vi "chooseOffensivePlay.vi"(8 "error in (no error)":errorcluster, 11 "Game in":refnum<class "Game.lvclass">) -> (0 "error out":errorcluster, 3 "Game out":refnum<class "Game.lvclass">)   [LabVIEW 2023, in "Game.lvclass"]
uses:
  Game.lvclass
  Referee_class/command_interpreted.ctl
  Game.lvclass/Game.ctl
  Team_class/Team.lvclass/Team.ctl
  Referee_class/Referee.lvclass/Referee.ctl
  StopOffensivePlay_class/StopOffensivePlay.lvclass
  PreparePenaltyEnemyPlay_class/PreparePenaltyEnemyPlay.lvclass
  EnemyPossessionAtEnemyFieldPlay_class/EnemyPossessionAtEnemyFieldPlay.lvclass
  EnemyPossessionAtOurFieldPlay_class/EnemyPossessionAtOurFieldPlay.lvclass
  PreparePenaltyAllyPlay_class/PreparePenaltyAllyPlay.lvclass
  KickPenaltyAllyPlay_class/KickPenaltyAllyPlay.lvclass
  PrepareKickoffAllyPlay_class/PrepareKickoffAllyPlay.lvclass
  PrepareKickoffEnemyPlay_class/PrepareKickoffEnemyPlay.lvclass
  SimplePass_class/SimplePass.lvclass
  PreparePassPlay_class/PreparePassPlay.lvclass
  PrepareRollToPassPlay_class/PrepareRollToPassPlay.lvclass
  PrepareDoublePassPlay_class/PrepareDoublePassPlay.lvclass
  PassToStriker_class/PassToStriker.lvclass
  C:/Users/roboi/Downloads/VSS_AI-Larc2023/Play_class/Play.lvclass
  PassTo2ndStriker_class/PassTo2ndStriker.lvclass
  TableWithStrikerPlay_class/TableWithStrikerPlay.lvclass
  TableWith2ndStrikerPlay_class/TableWith2ndStrikerPlay.lvclass
  DirectKickPlay_class/DirectKickPlay.lvclass
  DirectEnemyPlay_class/DirectEnemyPlay.lvclass
  NormalGamePlay_class/NormalGamePlay.lvclass
  TestPlay_class/TestPlay.lvclass
  BallOutOfFieldPlay_class/BallOutOfFieldPlay.lvclass
  Team_class/OffensivePlay.ctl
  Utilities_class/Utilities.lvclass
  Read OffensiveTeam.vi
  Read Referee.vi
  Referee_class/Read command_interpreted.vi
  Team_class/Read OffensivePlay.vi
  Team_class/Write OffensivePlay.vi
  Write OffensiveTeam.vi
  Ally_class/Ally.lvclass
  C:/Users/roboi/Downloads/VSS_AI-Larc2023/Team_class/Team.lvclass
  Referee_class/Referee.lvclass
  PassPlay_class/PassPlay.lvclass
  Play_class/Play.lvclass
panel:
  in  "Game in":refnum<class "Game.lvclass">
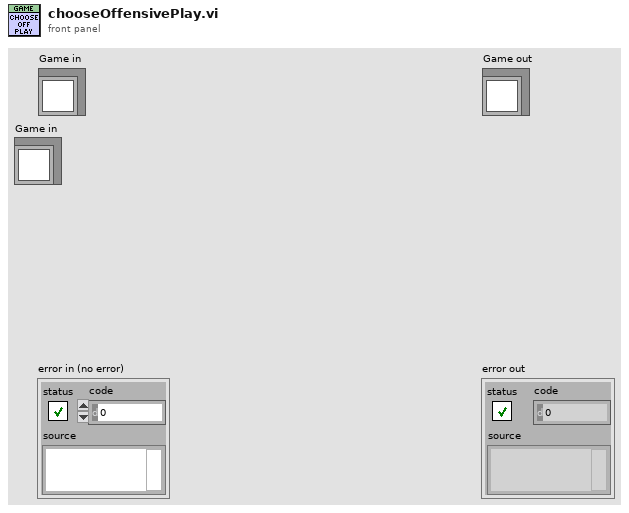
[diagram p1: front panel]
types:
  T1 = typedef "OffensivePlay.ctl" = enum16{"TableWithStriker", "TableWith2ndStrikerPlay", "PrepareDoublePass", "PrepareRollToPass", "SimplePass", "PreparePass", "PassToStriker", "BallOutOfField", "PassTo2ndStriker", "StopOffensive", "Prepare Penalty Enemy", "EnemyPossessionAtEnemyField", "EnemyPossesionAtOurField", "TestPlay", "PreparePenaltyAlly", "KickPenaltyAlly", "PrepareKickoffAlly", "PrepareKickoffEnemy", "IndirectEnemy", "DirectEnemy", "NormalGame", "DirectKick", "Pass", "Halt", "Timeout", "PassPlay", "PenaltyEnemy"}
  T2 = typedef "command_interpreted.ctl" = enum16{"Goal Ally", "Goal Enemy", "Ball Placement Enemy", "Ball Placement Ally", "Normal Half Time", "Extra Time  Break", "Extra Half Time", "None", "Post Game", "PKA Normal Start", "Prepare Kickoff Ally", "PKE Normal Start", "Prepare Kickoff Enemy", "Force Start", "Halt", "Timeout", "Prepare Penalty Ally", "Prepare Penalty Enemy", "PPA NormalStart", "PPE Normal Start", "Indirect Free Ally", "Direct Free Enemy", "Direct Free Ally", "Indirect Free Enemy", "Stop"}
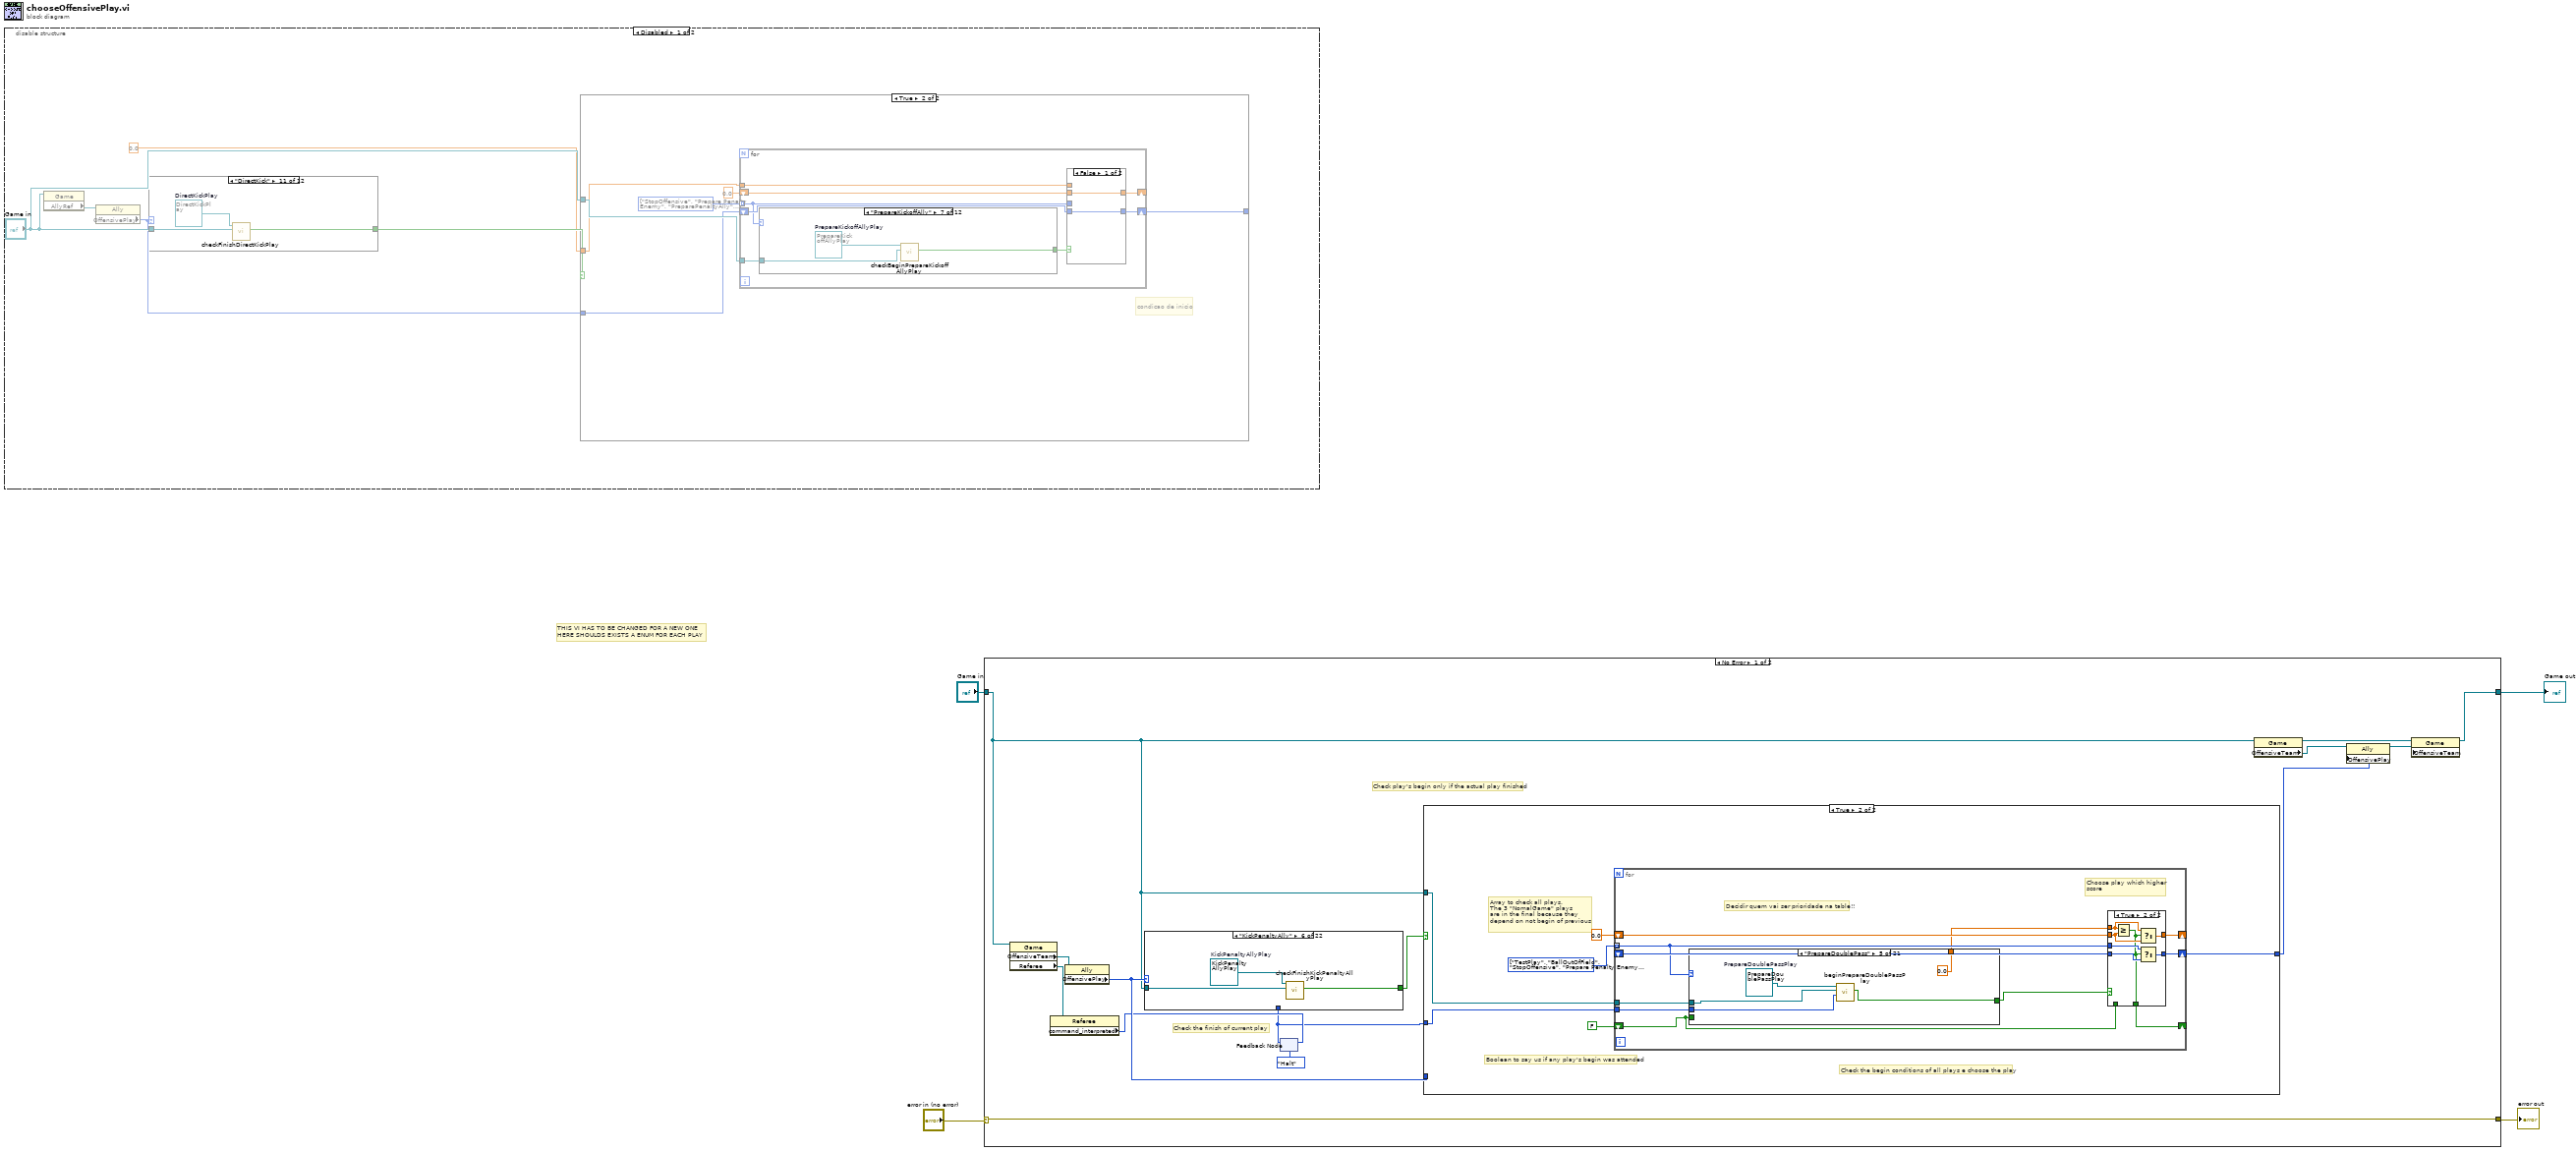
[diagram p0: block diagram]
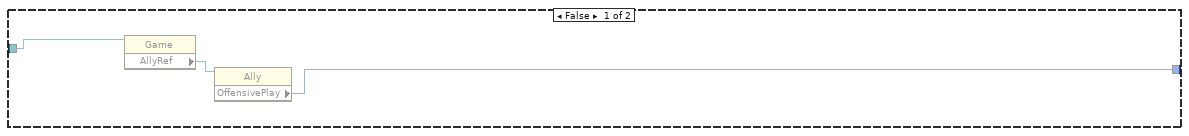
[diagram p2: hidden frame]
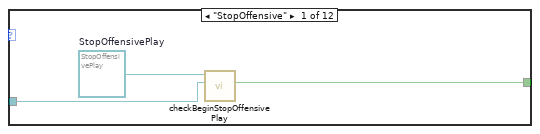
[diagram p3: hidden frame]
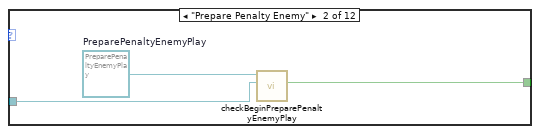
[diagram p4: hidden frame]
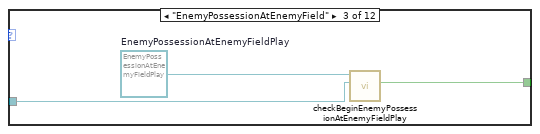
[diagram p5: hidden frame]
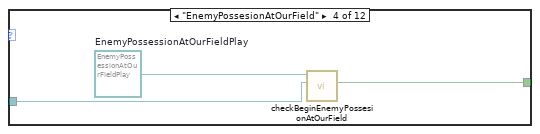
[diagram p6: hidden frame]
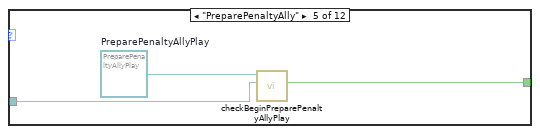
[diagram p7: hidden frame]
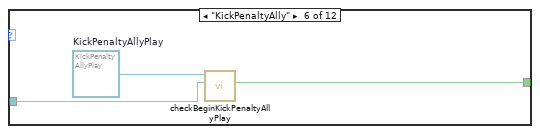
[diagram p8: hidden frame]
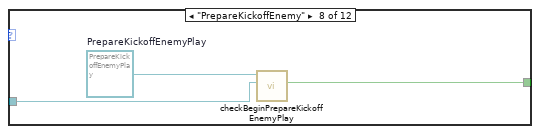
[diagram p9: hidden frame]
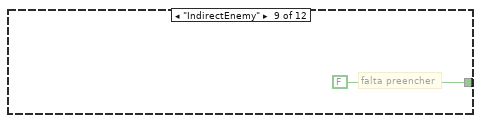
[diagram p10: hidden frame]
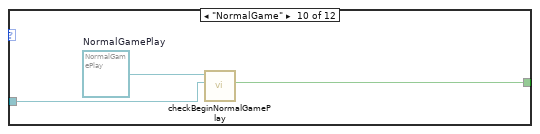
[diagram p11: hidden frame]
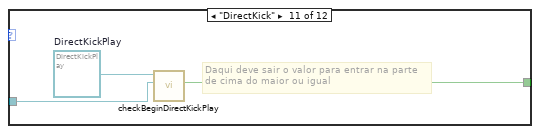
[diagram p12: hidden frame]
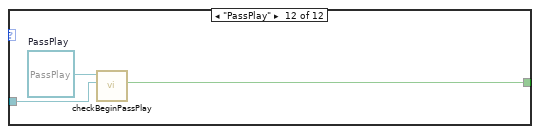
[diagram p13: hidden frame]
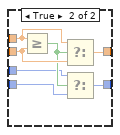
[diagram p14: hidden frame]
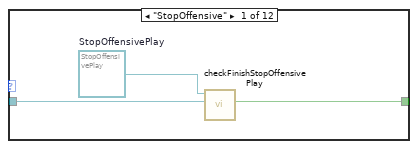
[diagram p15: hidden frame]
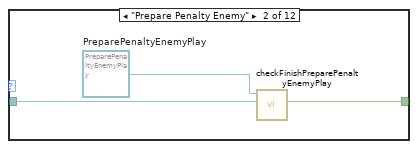
[diagram p16: hidden frame]
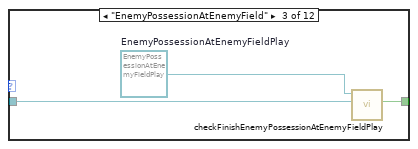
[diagram p17: hidden frame]
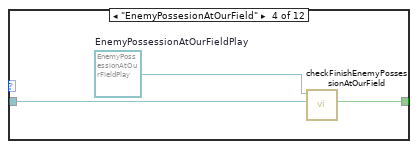
[diagram p18: hidden frame]
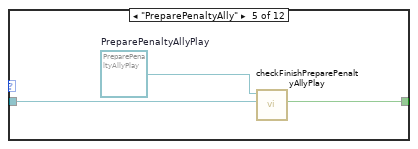
[diagram p19: hidden frame]
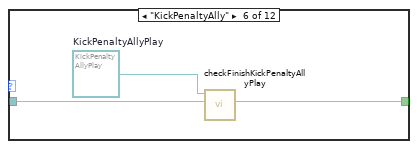
[diagram p20: hidden frame]
diagram:
  # "THIS VI HAS TO BE CHANGED FOR A NEW ONE\nHERE SHOULDS EXISTS A ENUM FOR EACH PLAY"
  n1 = disable-structure shown="Disabled" {
    frame Disabled {
      n2 = property class="Game"(reference="Game in") -> ("AllyRef"=w7:refnum<class "Ally.lvclass">)  [unwired: 1 in, 2 out]
      n3 = property class="Ally"(reference=w7) -> ("OffensivePlay"=w6:T1)  [unwired: 1 in, 2 out]
      n4 = case shown="\"DirectKick\"" w6 {
        tunnel: [w72 w74 w77 w80 w83 w86 w89 w92 FALSE w96 w99 w102] -> w9
        tunnel: "Game in" -> [w70 w75 w78 w81 w84 w87 w90 w93 _ w97 w100 w103]
        frame "StopOffensive" {
          w71 = refnum<class "StopOffensivePlay.lvclass"> refnum  # StopOffensivePlay
          n5 = call "checkFinishStopOffensivePlay.vi"("Game"=w70, "StopOffensivePlay in"=w71) -> ("Boolean"=w72:bool)  [unwired: 7 in, 2 out]
        }
        frame "Prepare Penalty Enemy" {
          w73 = refnum<class "PreparePenaltyEnemyPlay.lvclass"> refnum  # PreparePenaltyEnemyPlay
          n6 = call "checkFinishPreparePenaltyEnemyPlay.vi"("Game"=w75, "PreparePenaltyEnemyPlay in"=w73) -> ("Boolean"=w74:bool)  [unwired: 7 in, 2 out]
        }
        frame "EnemyPossessionAtEnemyField" {
          w76 = refnum<class "EnemyPossessionAtEnemyFieldPlay.lvclass"> refnum  # EnemyPossessionAtEnemyFieldPlay
          n7 = call "checkFinishEnemyPossessionAtEnemyFieldPlay.vi"("Game"=w78, "EnemyPossessionAtEnemyFieldPlay in"=w76) -> ("Boolean"=w77:bool)  [unwired: 7 in, 2 out]
        }
        frame "EnemyPossesionAtOurField" {
          w79 = refnum<class "EnemyPossessionAtOurFieldPlay.lvclass"> refnum  # EnemyPossessionAtOurFieldPlay
          n8 = call "checkFinishEnemyPossessionAtOurField.vi"("Game"=w81, "EnemyPossessionAtOurFieldPlay in"=w79) -> ("Boolean"=w80:bool)  [unwired: 7 in, 2 out]
        }
        frame "PreparePenaltyAlly" {
          w82 = refnum<class "PreparePenaltyAllyPlay.lvclass"> refnum  # PreparePenaltyAllyPlay
          n9 = call "checkFinishPreparePenaltyAllyPlay.vi"("Game"=w84, "PreparePenaltyAllyPlay in"=w82) -> ("Boolean"=w83:bool)  [unwired: 7 in, 2 out]
        }
        frame "KickPenaltyAlly" {
          w85 = refnum<class "KickPenaltyAllyPlay.lvclass"> refnum  # KickPenaltyAllyPlay
          n10 = call "checkFinishKickPenaltyAllyPlay.vi"("Game"=w87, "KickPenaltyAllyPlay in"=w85) -> ("Boolean"=w86:bool)  [unwired: 7 in, 2 out]
        }
        frame "PrepareKickoffAlly" {
          w88 = refnum<class "PrepareKickoffAllyPlay.lvclass"> refnum  # PrepareKickoffAllyPlay
          n11 = call "checkFinishPrepareKickoffAllyPlay.vi"("Game"=w90, "PrepareKickoffAllyPlay in"=w88) -> ("Boolean"=w89:bool)  [unwired: 7 in, 2 out]
        }
        frame "PrepareKickoffEnemy" {
          w91 = refnum<class "PrepareKickoffEnemyPlay.lvclass"> refnum  # PrepareKickoffEnemyPlay
          n12 = call "checkFinishPrepareKickoffEnemyPlay.vi"("Game"=w93, "PrepareKickoffEnemyPlay in"=w91) -> ("Boolean"=w92:bool)  [unwired: 7 in, 2 out]
        }
        frame "IndirectEnemy" {
          # "falta preencher"
        }
        frame "NormalGame" {
          w95 = refnum<class "NormalGamePlay.lvclass"> refnum  # NormalGamePlay
          n13 = call "checkFinishNormalGamePlay.vi"("Game"=w97, "NormalGamePlay in"=w95) -> ("Boolean"=w96:bool)  [unwired: 7 in, 2 out]
        }
        frame "DirectKick" {
          w98 = refnum<class "DirectKickPlay.lvclass"> refnum  # DirectKickPlay
          n14 = call "checkFinishDirectKickPlay.vi"("Game"=w100, "DirectKickPlay in"=w98) -> ("Boolean"=w99:bool)  [unwired: 7 in, 2 out]
        }
        frame "PassPlay" {
          w101 = refnum<class "PassPlay.lvclass"> refnum  # PassPlay
          n15 = call "checkFinishPassPlay.vi"("Game"=w103, "PassPlay in"=w101) -> ("Boolean"=w102:bool)  [unwired: 7 in, 2 out]
        }
      }
      n16 = case shown="True" w9 {
        tunnel: "Game in" -> [w12 w17]
        tunnel: w6 -> [_ w16]
        tunnel: 0.0 -> [_ w14]
        tunnel: [w10 w13] -> _
        frame False {
          n17 = property class="Game"(reference=w12) -> ("AllyRef"=w11:refnum<class "Ally.lvclass">)  [unwired: 1 in, 2 out]
          n18 = property class="Ally"(reference=w11) -> ("OffensivePlay"=w10:T1)  [unwired: 1 in, 2 out]
        }
        frame True {
          w18 = T1[] [enum."StopOffensive", enum."Prepare Penalty Enemy", enum."PreparePenaltyAlly", enum."KickPenaltyAlly", enum."PrepareKickoffAlly", enum."PrepareKickoffEnemy", enum."IndirectEnemy", enum."DirectKick", enum."PassPlay", enum."EnemyPossessionAtEnemyField", enum."EnemyPossesionAtOurField", enum."NormalGame"] items=["TableWithStriker", "TableWith2ndStrikerPlay", "PrepareDoublePass", "PrepareRollToPass", "SimplePass", "PreparePass", "PassToStriker", "BallOutOfField", "PassTo2ndStriker", "StopOffensive", "Prepare Penalty Enemy", "EnemyPossessionAtEnemyField", "EnemyPossesionAtOurField", "TestPlay", "PreparePenaltyAlly", "KickPenaltyAlly", "PrepareKickoffAlly", "PrepareKickoffEnemy", "IndirectEnemy", "DirectEnemy", "NormalGame", "DirectKick", "Pass", "Halt", "Timeout", "PassPlay", "PenaltyEnemy"] ("appended array")
          # "condicao de inicio"
          n19 = for {
            tunnel: w18 -> [w22] mode=indexing
            shift-right: [w25] -> _
            shift-left: 0.0 -> [w24]
            tunnel: w17 -> [w21]
            shift-right: [w23] -> w13
            shift-left: w16 -> [w26]
            tunnel: w14 -> [w19]
            n20 = case shown="\"PrepareKickoffAlly\"" w22 {
              tunnel: w21 -> [w29 w32 w35 w38 w41 w44 w47 w50 _ w54 w57 w60]
              tunnel: [w28 w31 w34 w37 w40 w43 w46 w49 FALSE w53 w56 w59] -> w20
              frame "StopOffensive" {
                w27 = refnum<class "StopOffensivePlay.lvclass"> refnum  # StopOffensivePlay
                n21 = call "checkBeginStopOffensivePlay.vi"("Game"=w29, "StopOffensivePlay in"=w27) -> ("Boolean"=w28:bool)  [unwired: 7 in, 2 out]
              }
              frame "Prepare Penalty Enemy" {
                w30 = refnum<class "PreparePenaltyEnemyPlay.lvclass"> refnum  # PreparePenaltyEnemyPlay
                n22 = call "checkBeginPreparePenaltyEnemyPlay.vi"("Game"=w32, "PreparePenaltyEnemyPlay in"=w30) -> ("Boolean"=w31:bool)  [unwired: 7 in, 2 out]
              }
              frame "EnemyPossessionAtEnemyField" {
                w33 = refnum<class "EnemyPossessionAtEnemyFieldPlay.lvclass"> refnum  # EnemyPossessionAtEnemyFieldPlay
                n23 = call "checkBeginEnemyPossessionAtEnemyFieldPlay.vi"("Game"=w35, "EnemyPossessionAtEnemyFieldPlay in"=w33) -> ("Begin?"=w34:bool)  [unwired: 7 in, 2 out]
              }
              frame "EnemyPossesionAtOurField" {
                w36 = refnum<class "EnemyPossessionAtOurFieldPlay.lvclass"> refnum  # EnemyPossessionAtOurFieldPlay
                n24 = call "checkBeginEnemyPossesionAtOurField.vi"("Game"=w38, "EnemyPossessionAtOurFieldPlay in"=w36) -> ("Begin?"=w37:bool)  [unwired: 7 in, 2 out]
              }
              frame "PreparePenaltyAlly" {
                w39 = refnum<class "PreparePenaltyAllyPlay.lvclass"> refnum  # PreparePenaltyAllyPlay
                n25 = call "checkBeginPreparePenaltyAllyPlay.vi"("Game"=w41, "PreparePenaltyAllyPlay in"=w39) -> ("Boolean"=w40:bool)  [unwired: 7 in, 2 out]
              }
              frame "KickPenaltyAlly" {
                w42 = refnum<class "KickPenaltyAllyPlay.lvclass"> refnum  # KickPenaltyAllyPlay
                n26 = call "checkBeginKickPenaltyAllyPlay.vi"("Game"=w44, "KickPenaltyAllyPlay in"=w42) -> ("Boolean"=w43:bool)  [unwired: 7 in, 2 out]
              }
              frame "PrepareKickoffAlly" {
                w45 = refnum<class "PrepareKickoffAllyPlay.lvclass"> refnum  # PrepareKickoffAllyPlay
                n27 = call "checkBeginPrepareKickoffAllyPlay.vi"("Game"=w47, "PrepareKickoffAllyPlay in"=w45) -> ("Boolean"=w46:bool)  [unwired: 7 in, 2 out]
              }
              frame "PrepareKickoffEnemy" {
                w48 = refnum<class "PrepareKickoffEnemyPlay.lvclass"> refnum  # PrepareKickoffEnemyPlay
                n28 = call "checkBeginPrepareKickoffEnemyPlay.vi"("Game"=w50, "PrepareKickoffEnemyPlay in"=w48) -> ("Boolean"=w49:bool)  [unwired: 7 in, 2 out]
              }
              frame "IndirectEnemy" {
                # "falta preencher"
              }
              frame "NormalGame" {
                w52 = refnum<class "NormalGamePlay.lvclass"> refnum  # NormalGamePlay
                n29 = call "checkBeginNormalGamePlay.vi"("Game"=w54, "NormalGamePlay in"=w52) -> ("Boolean"=w53:bool)  [unwired: 7 in, 2 out]
              }
              frame "DirectKick" {
                w55 = refnum<class "DirectKickPlay.lvclass"> refnum  # DirectKickPlay
                # "Daqui deve sair o valor para entrar na parte\nde cima do maior ou igual"
                n30 = call "checkBeginDirectKickPlay.vi"("Game"=w57, "DirectKickPlay in"=w55) -> ("Boolean"=w56:bool)  [unwired: 7 in, 2 out]
              }
              frame "PassPlay" {
                w58 = refnum<class "PassPlay.lvclass"> refnum  # PassPlay
                n31 = call "checkBeginPassPlay.vi"("Game"=w60, "PassPlay in"=w58) -> ("Boolean"=w59:bool)  [unwired: 7 in, 2 out]
              }
            }
            n32 = case shown="False" w20 {
              tunnel: w26 -> [w61 w63]
              tunnel: [w62 w69] -> w25
              tunnel: w24 -> [w62 w67]
              tunnel: w19 -> [_ w68]
              tunnel: w22 -> [_ w64]
              tunnel: [w61 w65] -> w23
              frame False {
              }
              frame True {
                n33 = Greater Or Equal?(x=w68, y=w67) -> (x >= y?=w66:bool)
                n34 = Select(t=w68, s=w66, f=w67) -> (s? t:f=w69:dbl)
                n35 = Select(t=w64, s=w66, f=w63) -> (s? t:f=w65:T1)
              }
            }
          }
        }
      }
    }
    frame Enabled {
    }
  }
  n36 = case shown="No Error" "error in (no error)" {
    selector: "error in (no error)" -> [w117 w328]
    tunnel: [w117 w328] -> w3
    tunnel: [w115 w327] -> w1
    tunnel: "Game in" -> [w105 w327]
    frame No Error {
      # "Check play's begin only if the actual play finished"
      # "Check the finish of current play"
      n37 = property class="Game"(reference=w105) -> ("OffensiveTeam"=w114:refnum<class "Ally.lvclass">, "Referee"=w110:refnum<class "Referee.lvclass">)  [unwired: 1 in, 2 out]
      n38 = property class="Referee"(reference=w110) -> ("command_interpreted"=w109:T2)  [unwired: 1 in, 2 out]
      n39 = property class="Ally"(reference=w114) -> ("OffensivePlay"=w111:T1)  [unwired: 1 in, 2 out]
      n40 = feedback-in #1(w109) -> ()
      n41 = feedback #1(command_interpreted."Halt" ("command_interpreted")) -> (w106:T2)
      n42 = case shown="\"KickPenaltyAlly\"" w111 {
        tunnel: [w118 w122 w126 w130 w134 w137 w141 w145 w149 w150 w154 w157 w159 w162 w165 w168 w171 w174 w179 TRUE w185 w188] -> w107
        tunnel: w105 -> [w119 w123 w127 w131 w135 w138 w142 w146 w147 w151 w155 w158 w160 w163 w166 w169 w172 w175 w178 w184 w186 w189]
        tunnel: w106 -> [_ _ w124 w128 w132 _ w139 w143 _ _ _ _ _ _ _ _ _ _ w177 w181 _ _]
        frame "StopOffensive" {
          w120 = refnum<class "StopOffensivePlay.lvclass"> refnum  # StopOffensivePlay
          n43 = call "checkFinishStopOffensivePlay.vi"("Game"=w119, "StopOffensivePlay in"=w120) -> ("Boolean"=w118:bool)  [unwired: 7 in, 2 out]
        }
        frame "Prepare Penalty Enemy" {
          w121 = refnum<class "PreparePenaltyEnemyPlay.lvclass"> refnum  # PreparePenaltyEnemyPlay
          n44 = call "checkFinishPreparePenaltyEnemyPlay.vi"("Game"=w123, "PreparePenaltyEnemyPlay in"=w121) -> ("Boolean"=w122:bool)  [unwired: 7 in, 2 out]
        }
        frame "EnemyPossessionAtEnemyField" {
          w125 = refnum<class "EnemyPossessionAtEnemyFieldPlay.lvclass"> refnum  # EnemyPossessionAtEnemyFieldPlay
          n45 = call "checkFinishEnemyPossessionAtEnemyFieldPlay.vi"("last command_interpreted"=w124, "Game"=w127, "EnemyPossessionAtEnemyFieldPlay in"=w125) -> ("Boolean"=w126:bool)  [unwired: 6 in, 2 out]
        }
        frame "EnemyPossesionAtOurField" {
          w129 = refnum<class "EnemyPossessionAtOurFieldPlay.lvclass"> refnum  # EnemyPossessionAtOurFieldPlay
          n46 = call "checkFinishEnemyPossessionAtOurField.vi"("last command_interpreted"=w128, "Game"=w131, "EnemyPossessionAtOurFieldPlay in"=w129) -> ("Boolean"=w130:bool)  [unwired: 6 in, 2 out]
        }
        frame "PreparePenaltyAlly" {
          w133 = refnum<class "PreparePenaltyAllyPlay.lvclass"> refnum  # PreparePenaltyAllyPlay
          n47 = call "checkFinishPreparePenaltyAllyPlay.vi"("last command_interpreted"=w132, "Game"=w135, "PreparePenaltyAllyPlay in"=w133) -> ("Boolean"=w134:bool)  [unwired: 6 in, 2 out]
        }
        frame "KickPenaltyAlly" {
          w136 = refnum<class "KickPenaltyAllyPlay.lvclass"> refnum  # KickPenaltyAllyPlay
          n48 = call "checkFinishKickPenaltyAllyPlay.vi"("Game"=w138, "KickPenaltyAllyPlay in"=w136) -> ("Boolean"=w137:bool)  [unwired: 7 in, 2 out]
        }
        frame "PrepareKickoffAlly" {
          w140 = refnum<class "PrepareKickoffAllyPlay.lvclass"> refnum  # PrepareKickoffAllyPlay
          n49 = call "checkFinishPrepareKickoffAllyPlay.vi"("last command_interpreted"=w139, "Game"=w142, "PrepareKickoffAllyPlay in"=w140) -> ("Boolean"=w141:bool)  [unwired: 6 in, 2 out]
        }
        frame "PrepareKickoffEnemy" {
          w144 = refnum<class "PrepareKickoffEnemyPlay.lvclass"> refnum  # PrepareKickoffEnemyPlay
          n50 = call "checkFinishPrepareKickoffEnemyPlay.vi"("last command_interpreted"=w143, "Game"=w146, "PrepareKickoffEnemyPlay in"=w144) -> ("Boolean"=w145:bool)  [unwired: 6 in, 2 out]
        }
        frame "SimplePass" {
          w148 = refnum<class "SimplePass.lvclass"> refnum  # SimplePass in
          n51 = call "finishSimplePassPlay.vi"("Game in"=w147, "SimplePass in"=w148) -> ("finishSimplePass?"=w149:bool)  [unwired: 7 in, 2 out]
        }
        frame "PreparePass" {
          w152 = refnum<class "PreparePassPlay.lvclass"> refnum  # PreparePassPlay
          n52 = call "finishPreparePassPlay.vi"("Game"=w151, "PreparePassPlay in"=w152) -> ("FinishPreparePass?"=w150:bool)  [unwired: 7 in, 2 out]
        }
        frame "PrepareRollToPass" {
          w153 = refnum<class "PrepareRollToPassPlay.lvclass"> refnum  # PrepareRollToPassPlay in
          n53 = call "finishPrepareRollToPassPlay.vi"("Game"=w155, "PrepareRollToPassPlay in"=w153) -> ("FinishPrepareRollToPass?"=w154:bool)  [unwired: 7 in, 2 out]
        }
        frame "PrepareDoublePass" {
          w156 = refnum<class "PrepareDoublePassPlay.lvclass"> refnum  # PrepareDoublePassPlay
          n54 = call "finishPrepareDoublePassPlay.vi"("Game"=w158, "PrepareDoublePassPlay in"=w156) -> ("FinishPrepareDoublePass?"=w157:bool)  [unwired: 7 in, 2 out]
        }
        frame "PassToStriker" {
          w161 = refnum<class "PassToStriker.lvclass"> refnum  # PassToStriker
          n55 = call "finishPassToStrikerPlay.vi"("Game"=w160, "PassToStriker in"=w161) -> ("result"=w159:bool)  [unwired: 7 in, 2 out]
        }
        frame "PassTo2ndStriker" {
          w164 = refnum<class "PassTo2ndStriker.lvclass"> refnum  # PassTo2ndStriker
          n56 = call "finishPassTo2ndStrikerPlay.vi"("Game"=w163, "PassTo2ndStriker in"=w164) -> ("value"=w162:bool)  [unwired: 7 in, 2 out]
        }
        frame "TableWithStriker" {
          w167 = refnum<class "TableWithStrikerPlay.lvclass"> refnum  # TableWith2ndStrikerPlay
          n57 = call "finishTableWithStrikerPlay.vi"("Game"=w166, "TableWithStrikerPlay in"=w167) -> ("finishTableWith2ndStriker?"=w165:bool)  [unwired: 8 in, 1 out]
        }
        frame "TableWith2ndStrikerPlay" {
          w170 = refnum<class "TableWith2ndStrikerPlay.lvclass"> refnum  # TableWith2ndStrikerPlay
          n58 = call "finishTableWith2ndStrikerPlay.vi"("Game"=w169, "TableWith2ndStrikerPlay in"=w170) -> ("finishTableWith2ndStriker?"=w168:bool)  [unwired: 8 in, 1 out]
        }
        frame "IndirectEnemy" {
          w173 = refnum<class "TableWithStrikerPlay.lvclass"> refnum  # TableWith2ndStrikerPlay
          n59 = call "finishTableWithStrikerPlay.vi"("Game"=w172, "TableWithStrikerPlay in"=w173) -> ("finishTableWith2ndStriker?"=w171:bool)  [unwired: 8 in, 1 out]
        }
        frame "DirectKick" {
          w176 = refnum<class "DirectKickPlay.lvclass"> refnum  # DirectKickPlay
          n60 = call "finishDirectKickPlay.vi"("Game"=w175, "DirectKickPlay in"=w176) -> ("result"=w174:bool)  [unwired: 7 in, 2 out]
        }
        frame "DirectEnemy" {
          w180 = refnum<class "DirectEnemyPlay.lvclass"> refnum  # DirectEnemyPlay
          n61 = call "checkFinishDirectEnemyPlay.vi"("last command_interpreted"=w177, "Game"=w178, "DirectEnemyPlay in"=w180) -> ("Boolean"=w179:bool)  [unwired: 6 in, 2 out]
        }
        frame "NormalGame", Default {
          w183 = refnum<class "NormalGamePlay.lvclass"> refnum  # NormalGamePlay
          n62 = call "checkFinishNormalGamePlay.vi"("last command_interpreted"=w181, "Game"=w184, "NormalGamePlay in"=w183) -> ()  [unwired: 6 in, 3 out]
        }
        frame "TestPlay" {
          w187 = refnum<class "TestPlay.lvclass"> refnum  # TestPlay
          n63 = call "checkFinishTestPlay.vi"("Game"=w186, "TestPlay in"=w187) -> ("Boolean"=w185:bool)  [unwired: 7 in, 2 out]
        }
        frame "BallOutOfField" {
          w190 = refnum<class "BallOutOfFieldPlay.lvclass"> refnum  # BallOutOfFieldPlay
          n64 = call "checkFinishBallOutOfFieldPlay.vi"("Game"=w189, "BallOutOfFieldPlay in"=w190) -> ("Finish Ball Out?"=w188:bool)  [unwired: 7 in, 2 out]
        }
      }
      n65 = case shown="True" w107 {
        tunnel: w111 -> [w191 _]
        tunnel: w105 -> [_ w197]
        tunnel: [w191 w196] -> w104
        tunnel: w106 -> [_ w192]
        frame False {
        }
        frame True {
          w193 = T1[] [enum."TestPlay", enum."BallOutOfField", enum."StopOffensive", enum."Prepare Penalty Enemy", enum."PreparePenaltyAlly", enum."KickPenaltyAlly", enum."PrepareKickoffAlly", enum."PrepareKickoffEnemy", enum."DirectEnemy", enum."SimplePass", enum."PreparePass", enum."PrepareRollToPass", enum."PrepareDoublePass", enum."PassToStriker", enum."PassTo2ndStriker", enum."TableWithStriker", enum."TableWith2ndStrikerPlay", enum."DirectKick", enum."EnemyPossesionAtOurField", enum."EnemyPossessionAtEnemyField", enum."NormalGame"] items=["TableWithStriker", "TableWith2ndStrikerPlay", "PrepareDoublePass", "PrepareRollToPass", "SimplePass", "PreparePass", "PassToStriker", "BallOutOfField", "PassTo2ndStriker", "StopOffensive", "Prepare Penalty Enemy", "EnemyPossessionAtEnemyField", "EnemyPossesionAtOurField", "TestPlay", "PreparePenaltyAlly", "KickPenaltyAlly", "PrepareKickoffAlly", "PrepareKickoffEnemy", "IndirectEnemy", "DirectEnemy", "NormalGame", "DirectKick", "Pass", "Halt", "Timeout", "PassPlay", "PenaltyEnemy"] ("output array")
          # "Boolean to say us if any play's begin was attended"
          # "Array to check all plays.\nThe 3 \"NomalGame\" plays\nare in the final because they\ndepend on not begin of previous"
          # "Check the begin conditions of all plays e choose the play"
          n66 = for {
            tunnel: w193 -> [w204] mode=indexing
            shift-right: [w207] -> _
            shift-left: 0.0 -> [w206]
            tunnel: w197 -> [w203]
            shift-right: [w205] -> w196
            shift-left: _ -> [w208]
            shift-right: [w201] -> _
            shift-left: FALSE -> [w199]
            tunnel: w192 -> [w198]
            # "Decidir quem vai ser prioridade na table!!"
            # "Choose play which higher\nscore"
            n67 = case shown="\"PrepareDoublePass\"" w204 {
              selector: w204 -> [_ _ _ _ _ w233 w240 w248 w255 _ _ _ _ _ _ _ _ _ _ _ _]
              tunnel: w203 -> [w211 w215 w221 w224 w229 w237 w243 w249 w256 w261 w266 w271 w278 w285 w290 w294 w299 w304 w307 _ w315]
              tunnel: [w210 w217 w220 w227 w232 w239 w245 w251 w257 w260 w265 w270 w272 w282 w289 w293 w298 w303 w306 w311 w314] -> w200
              tunnel: [1.0 ("Score out") 2.0 1.0 1.0 0.0 w235 w241 w250 w253 1.0 0.0 0.0 0.0 0.0 0.0 0.0 0.0 0.0 0.0 0.0 w313] -> w202
              tunnel: w199 -> [_ _ _ _ _ _ _ _ _ _ _ _ w273 w279 _ _ _ _ _ w310 _]
              tunnel: w198 -> [_ w213 w218 w223 w230 _ _ _ _ _ _ w267 _ _ w286 _ w295 w300 w305 _ _]
              frame "BallOutOfField" {
                w212 = refnum<class "BallOutOfFieldPlay.lvclass"> refnum  # BallOutOfFieldPlay
                n68 = call "checkBeginBallOutOfFieldPlay.vi"("Game"=w211, "BallOutOfFieldPlay in"=w212) -> ("ball_out"=w210:bool)  [unwired: 7 in, 2 out]
              }
              frame "SimplePass" {
                w214 = refnum<class "SimplePass.lvclass"> refnum  # SimplePass in
                n69 = call "beginSimplePassPlay.vi"("last command_interpreted"=w213, "Game in"=w215, "SimplePass in"=w214) -> ("BeginSimplePass?"=w217:bool)  [unwired: 6 in, 2 out]
              }
              frame "PreparePass" {
                w222 = refnum<class "PreparePassPlay.lvclass"> refnum  # PreparePassPlay
                n70 = call "beginPreparePassPlay.vi"("last command_interpreted"=w218, "Game"=w221, "PreparePassPlay in"=w222) -> ("BeginPreparePass?"=w220:bool)  [unwired: 6 in, 2 out]
              }
              frame "PrepareRollToPass" {
                w225 = refnum<class "PrepareRollToPassPlay.lvclass"> refnum  # PrepareRollToPassPlay in
                n71 = call "beginPrepareRollToPassPlay.vi"("last command_interpreted"=w223, "Game"=w224, "PrepareRollToPassPlay in"=w225) -> ("BeginPrepareRollToPass?"=w227:bool)  [unwired: 6 in, 2 out]
              }
              frame "PrepareDoublePass" {
                w228 = refnum<class "PrepareDoublePassPlay.lvclass"> refnum  # PrepareDoublePassPlay
                n72 = call "beginPrepareDoublePassPlay.vi"("last command_interpreted"=w230, "Game"=w229, "PrepareDoublePassPlay in"=w228) -> ("BeginPrepareDoublePass?"=w232:bool)  [unwired: 7 in, 1 out]
              }
              frame "PassToStriker" {
                w238 = refnum<class "PassToStriker.lvclass"> refnum  # PassToStriker
                n73 = call "beginPassToStrikerPlay.vi"("Game"=w237, "PassToStriker in"=w238) -> ("BeginPassToStriker?"=w239:bool, "PassToStriker out"=w234:refnum<class "PassToStriker.lvclass">)  [unwired: 7 in, 1 out]
                n74 = call "ChoosePass.vi"("OffensivePlay"=w233, "Stk/2ndStk"=enum16{"Striker", "2ndStriker"}."Striker", "Game"=w237, "Play in"=w234) -> ("Factor Pass"=w235:dbl)  [unwired: 5 in, 2 out]
              }
              frame "PassTo2ndStriker" {
                w246 = refnum<class "PassTo2ndStriker.lvclass"> refnum  # PassTo2ndStriker
                n75 = call "beginPassTo2ndStrikerPlay.vi"("Game"=w243, "PassTo2ndStriker in"=w246) -> ("result"=w245:bool, "PassTo2ndStriker out"=w244:refnum<class "PassTo2ndStriker.lvclass">)  [unwired: 7 in, 1 out]
                n76 = call "ChoosePass.vi"("OffensivePlay"=w240, "Stk/2ndStk"=enum16{"Striker", "2ndStriker"}."2ndStriker", "Game"=w243, "Play in"=w244) -> ("Factor Pass"=w241:dbl)  [unwired: 5 in, 2 out]
              }
              frame "TableWithStriker" {
                w252 = refnum<class "TableWithStrikerPlay.lvclass"> refnum  # TableWith2ndStrikerPlay
                n77 = call "beginTableWithStrikerPlay.vi"("Game"=w249, "TableWithStrikerPlay in"=w252) -> ("BeginTableWithStriker?"=w251:bool)  [unwired: 8 in, 1 out]
                n78 = call-dynamic "FactorPass.vi"("OffensivePlay"=w248, "Game"=w249, "Utilities in"=refnum<class "Utilities.lvclass"> refnum) -> ("Critério de marcação Normalizado"=w250:dbl)  [unwired: 6 in, 2 out]
              }
              frame "TableWith2ndStrikerPlay" {
                w258 = refnum<class "TableWith2ndStrikerPlay.lvclass"> refnum  # TableWith2ndStrikerPlay
                n79 = call "beginTableWith2ndStikerPlay.vi"("Game"=w256, "TableWith2ndStrikerPlay in"=w258) -> ("BeginTableWith2ndStriker?"=w257:bool)  [unwired: 7 in, 2 out]
                n80 = call-dynamic "FactorPass.vi"("OffensivePlay"=w255, "Game"=w256, "Utilities in"=refnum<class "Utilities.lvclass"> refnum) -> ("Critério de marcação Normalizado"=w253:dbl)  [unwired: 6 in, 2 out]
              }
              frame "DirectKick" {
                w262 = refnum<class "DirectKickPlay.lvclass"> refnum  # DirectKickPlay
                n81 = call "beginDirectKickPlay.vi"("Game"=w261, "DirectKickPlay in"=w262) -> ("beginDirectKick?"=w260:bool)  [unwired: 7 in, 2 out]
              }
              frame "StopOffensive" {
                w264 = refnum<class "StopOffensivePlay.lvclass"> refnum  # StopOffensivePlay
                n82 = call "checkBeginStopOffensivePlay.vi"("Game"=w266, "StopOffensivePlay in"=w264) -> ("Boolean"=w265:bool)  [unwired: 7 in, 2 out]
              }
              frame "Prepare Penalty Enemy" {
                w269 = refnum<class "PreparePenaltyEnemyPlay.lvclass"> refnum  # PreparePenaltyEnemyPlay
                n83 = call "checkBeginPreparePenaltyEnemyPlay.vi"("last command_interpreted"=w267, "Game"=w271, "PreparePenaltyEnemyPlay in"=w269) -> ("Boolean"=w270:bool)  [unwired: 6 in, 2 out]
              }
              frame "EnemyPossessionAtEnemyField" {
                w277 = refnum<class "EnemyPossessionAtEnemyFieldPlay.lvclass"> refnum  # EnemyPossessionAtEnemyFieldPlay
                n84 = call "checkBeginEnemyPossessionAtEnemyFieldPlay.vi"("Game"=w278, "EnemyPossessionAtEnemyFieldPlay in"=w277) -> ("Begin?"=w275:bool)  [unwired: 7 in, 2 out]
                n85 = Not(x=w273) -> (.not. x?=w274:bool)
                n86 = And(x=w275, y=w274) -> (x .and. y?=w272:bool)
              }
              frame "EnemyPossesionAtOurField" {
                w284 = refnum<class "EnemyPossessionAtOurFieldPlay.lvclass"> refnum  # EnemyPossessionAtOurFieldPlay
                n87 = call "checkBeginEnemyPossesionAtOurField.vi"("Game"=w285, "EnemyPossessionAtOurFieldPlay in"=w284) -> ("Begin?"=w281:bool)  [unwired: 7 in, 2 out]
                n88 = Not(x=w279) -> (.not. x?=w280:bool)
                n89 = And(x=w281, y=w280) -> (x .and. y?=w282:bool)
              }
              frame "PreparePenaltyAlly" {
                w288 = refnum<class "PreparePenaltyAllyPlay.lvclass"> refnum  # PreparePenaltyAllyPlay
                n90 = call "checkBeginPreparePenaltyAllyPlay.vi"("last command_interpreted"=w286, "Game"=w290, "PreparePenaltyAllyPlay in"=w288) -> ("Boolean"=w289:bool)  [unwired: 6 in, 2 out]
              }
              frame "KickPenaltyAlly" {
                w292 = refnum<class "KickPenaltyAllyPlay.lvclass"> refnum  # KickPenaltyAllyPlay
                n91 = call "checkBeginKickPenaltyAllyPlay.vi"("Game"=w294, "KickPenaltyAllyPlay in"=w292) -> ("Boolean"=w293:bool)  [unwired: 7 in, 2 out]
              }
              frame "PrepareKickoffAlly" {
                w297 = refnum<class "PrepareKickoffAllyPlay.lvclass"> refnum  # PrepareKickoffAllyPlay
                n92 = call "checkBeginPrepareKickoffAllyPlay.vi"("last command_interpreted"=w295, "Game"=w299, "PrepareKickoffAllyPlay in"=w297) -> ("Boolean"=w298:bool)  [unwired: 6 in, 2 out]
              }
              frame "PrepareKickoffEnemy" {
                w302 = refnum<class "PrepareKickoffEnemyPlay.lvclass"> refnum  # PrepareKickoffEnemyPlay
                n93 = call "checkBeginPrepareKickoffEnemyPlay.vi"("last command_interpreted"=w300, "Game"=w304, "PrepareKickoffEnemyPlay in"=w302) -> ("Boolean"=w303:bool)  [unwired: 6 in, 2 out]
              }
              frame "DirectEnemy" {
                w308 = refnum<class "DirectEnemyPlay.lvclass"> refnum  # DirectEnemyPlay
                n94 = call "checkBeginDirectEnemyPlay.vi"("last command_interpreted"=w305, "Game"=w307, "DirectEnemyPlay in"=w308) -> ("Boolean"=w306:bool)  [unwired: 6 in, 2 out]
              }
              frame "NormalGame", Default {
                n95 = Not(x=w310) -> (.not. x?=w311:bool)
              }
              frame "TestPlay" {
                w316 = refnum<class "TestPlay.lvclass"> refnum  # TestPlay
                n96 = call "checkBeginTestPlay.vi"("Game"=w315, "TestPlay in"=w316) -> ("Test"=w314:bool, "Score out"=w313:dbl)  [unwired: 6 in, 2 out]
              }
            }
            n97 = case shown="True" w200 {
              tunnel: w208 -> [w318 w321]
              tunnel: [w319 w326] -> w207
              tunnel: w206 -> [w319 w324]
              tunnel: w202 -> [_ w325]
              tunnel: w204 -> [_ w322]
              tunnel: [w318 w323] -> w205
              tunnel: [w317 w320] -> w201
              tunnel: w199 -> [w317 _]
              frame False {
              }
              frame True {
                n98 = Greater Or Equal?(x=w325, y=w324) -> (x >= y?=w320:bool)
                n99 = Select(t=w325, s=w320, f=w324) -> (s? t:f=w326:dbl)
                n100 = Select(t=w322, s=w320, f=w321) -> (s? t:f=w323:T1)
              }
            }
          }
        }
      }
      n101 = property class="Game"(reference=w105) -> (reference out=w116:refnum<class "Game.lvclass">, "OffensiveTeam"=w113:refnum<class "Ally.lvclass">)  [unwired: 1 in, 1 out]
      n102 = property class="Ally"(reference=w113, "OffensivePlay"=w104) -> (reference out=w112:refnum<class "Ally.lvclass">)  [unwired: 1 in, 1 out]
      n103 = property class="Game"(reference=w116, "OffensiveTeam"=w112) -> (reference out=w115:refnum<class "Game.lvclass">)  [unwired: 1 in, 1 out]
    }
    frame Error {
    }
  }
  "error out" <- w3
  "Game out" <- w1
